vi "MT Detect ASK.vi"(5 "input complex waveform":T3={"t0"=0.0, "dt"=1.0, "Y"=[]} {"Y" format="%.3f"; "dt" format="%^.2e"; "t0" format="%.4f"}, 7 "ASK system parameters":T2={"samples per symbol (16)"=16, "symbol map"=[]} {"symbol map" format="%.3f"}, 9 "synchronization parameters":T1 {"sync sequence" format="%.2f"}, 11 "error in (no error)":errorcluster, 12 "matched filter coefficients":dbl[](array[numeric]) format="%.2f", 13 "reset? (T)":bool=TRUE, 14 "flush buffers? (F)":bool) -> (6 "output bit stream":i8[](array[numeric]), 10 "sync found index (symbols)":dbl format="%.4f", 15 "error out":errorcluster)   [LabVIEW 2020, in "niDMT.lvlib"]
doc: "Demodulates an amplitude-shift keying (ASK)-modulated complex baseband waveform and returns the demodulated bit stream. This VI attempts to remove carrier and phase offset by locking to the carrier signal."
uses:
  <vilib>/addons/Modulation/niDMT.lvlib
  <vilib>/addons/Modulation/Analog/controls/Complex Data Waveform.ctl
  <vilib>/Utility/error.llb/Error Cluster From Error Code.vi
  <vilib>/addons/Modulation/Digital/Support/Common/mod_Truncate FIR Filter (complex).vi
  <vilib>/addons/Modulation/niAMT.lvlib
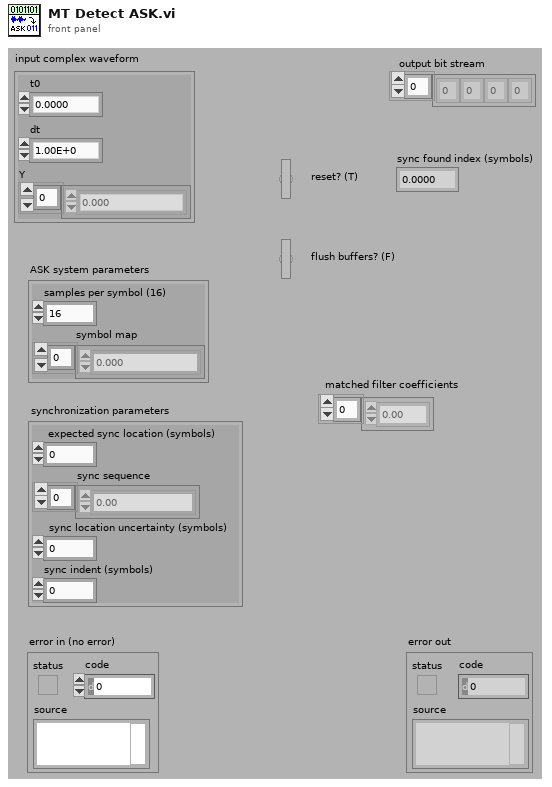
[diagram p1: front panel]
types:
  T1 = cluster{"expected sync location (symbols)":i32, "sync sequence":cdb[], "sync location uncertainty (symbols)":i32, "sync indent (symbols)":i32}
  T2 = cluster{"samples per symbol (16)":i32, "symbol map":cdb[]}
  T3 = typedef "niAMT.lvlib/Complex Data Waveform.ctl" = cluster{"t0":dbl, "dt":dbl, "Y":cdb[]}
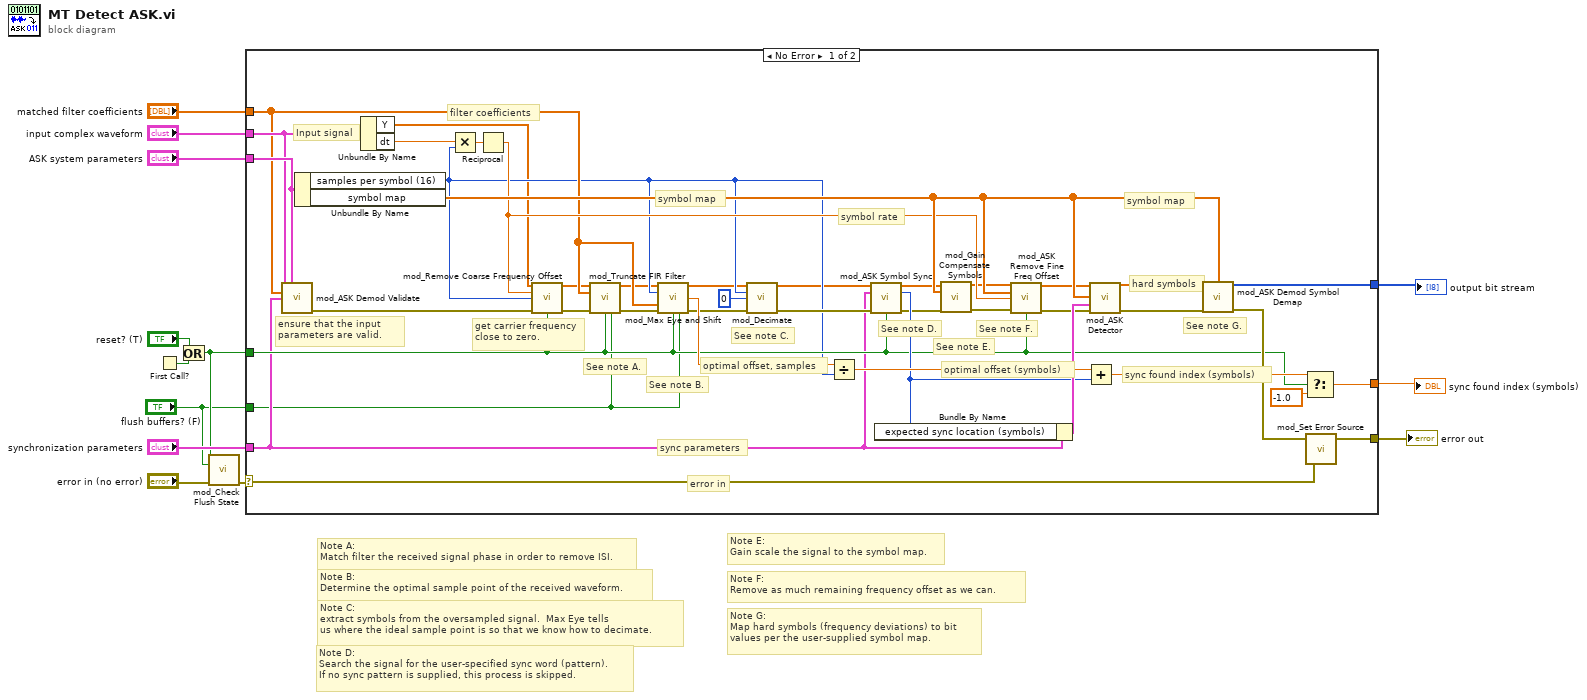
[diagram p0: block diagram]
diagram:
  # "Note E:\nGain scale the signal to the symbol map."
  # "Note G:\nMap hard symbols (frequency deviations) to bit\nvalues per the user-supplied symbol map."
  # "Note D:\nSearch the signal for the user-specified sync word (pattern).\nIf no sync pattern is supplied, this process is skipped."
  # "Note F:\nRemove as much remaining frequency offset as we can."
  # "Note C:\nextract symbols from the oversampled signal.  Max Eye tells\nus where the ideal sample point is so that we know how to decimate."
  # "Note B:\nDetermine the optimal sample point of the received waveform."
  # "Note A:\nMatch filter the received signal phase in order to remove ISI."
  n1 = First Call?() -> (First Call?: T/F=w6:bool)
  n2 = Or(x="reset? (T)", y=w6) -> (x .or. y?=w2:bool)
  n3 = call <vilib>:"mod_Check Flush State.vi"("reset?"=w2, "flush buffers? (F)"="flush buffers? (F)", "error in (no error)"="error in (no error)") -> ("error out"=w4:errorcluster)  [unwired: 12 out]
  n4 = case shown="No Error" w4 {
    selector: w4 -> [w35 w55]
    tunnel: w2 -> [w28 _]
    tunnel: "input complex waveform" -> [w39 _]
    tunnel: [w34 w55] -> w7
    tunnel: "matched filter coefficients" -> [w25 _]
    tunnel: [w54 _] -> w9
    tunnel: [w40 _] -> w8
    tunnel: "ASK system parameters" -> [w51 _]
    tunnel: "synchronization parameters" -> [w22 _]
    tunnel: "flush buffers? (F)" -> [w21 _]
    frame No Error {
      # "filter coefficients"
      # "error in"
      # "Input signal"
      # "sync found index (symbols)"
      # "symbol rate"
      # "hard symbols"
      # "symbol map"
      # "sync parameters"
      # "error in"
      # "symbol map"
      # "See note E."
      # "See note G."
      # "See note D."
      # "See note F."
      # "See note C."
      # "get carrier frequency close to zero."
      # "ensure that the input parameters are valid."
      # "See note B."
      # "See note A."
      # "optimal offset (symbols)"
      # "optimal offset, samples"
      n5 = call <vilib>:"mod_ASK Demod Validate.vi"("Input Complex Waveform"=w39, "PAM System Parameters"=w51, "Matched Filter Coefficients"=w25, "Synchronization Parameters"=w22) -> ("error out"=w45:errorcluster)  [unwired: 11 out]
      n6 = Unbundle By Name(w51) -> ("samples per symbol (16)"=w23:i32, "symbol map"=w31:cdb[])
      n7 = Unbundle By Name(w39) -> ("Y"=w20:cdb[], "dt"=w48:dbl)
      n8 = Multiply(x=w48, y=w23) -> (x*y=w49:dbl)
      n9 = Reciprocal(x=w49) -> (1/x=w29:dbl)
      n10 = call <vilib>:"mod_Remove Coarse Frequency Offset.vi"("Signal In"=w20, "Symbol Rate, Hz"=w29, "Samples Per Symbol (16)"=w23, "error in (no error)"=w45, "Reset? (T)"=w28) -> ("Signal Out"=w19:cdb[], "error out"=w53:errorcluster)  [unwired: 9 out]
      n11 = call-poly <vilib>:"mod_Truncate FIR Filter.vi"("Signal In"=w19, "Filter Coefficients"=w25, "error in (no error)"=w53, "Reset? (T)"=w28, "flush buffers? (F)"=w21) -> ("Signal Out"=w18:cdb[], "error out"=w46:errorcluster)  [unwired: 7 in, 2 out]
      n12 = call <vilib>:"mod_Max Eye and Shift.vi"("Signal In"=w18, "Samples Per Symbol (16)"=w23, "matched filter coefficients"=w25, "error in (no error)"=w46, "Reset? (T)"=w28, "flush buffers? (F)"=w21) -> ("Signal Out"=w17:cdb[], "Optimal Offset (in Samples)"=w38:dbl, "error out"=w24:errorcluster)  [unwired: 1 in, 6 out]
      n13 = call <vilib>:"mod_Decimate.vi"("Signal In"=w17, "Samples Per Symbol (16)"=w23, "Offset"=0, "error in (no error)"=w24) -> ("Signal Out"=w16:cdb[], "error out"=w50:errorcluster)  [unwired: 1 in, 9 out]
      n14 = Divide(x=w38, y=w23) -> (x/y=w47:dbl)
      n15 = call <vilib>:"mod_ASK Symbol Sync.vi"("Signal In"=w16, "Synchronization Parameters"=w22, "error in (no error)"=w50, "Reset? (T)"=w28) -> ("Signal Out"=w15:cdb[], "Sync Location (symbols)"=w44:i32, "error out"=w33:errorcluster)  [unwired: 9 out]
      n16 = Bundle By Name(cluster=w22, "expected sync location (symbols)"=w44) -> (w52:T1)
      n17 = call <vilib>:"mod_Gain Compensate Symbols.vi"("Symbols In"=w15, "Symbol Map"=w31, "error in (no error)"=w33) -> ("Symbols Out"=w14:cdb[], "error out"=w32:errorcluster)  [unwired: 11 out]
      n18 = call <vilib>:"mod_ASK Remove Fine Freq Offset.vi"("Symbols"=w14, "Symbol Map"=w31, "Symbol Rate, Hz"=w29, "error in (no error)"=w32, "Reset? (T)"=w28) -> ("Symbols"=w30:cdb[], "error out"=w43:errorcluster)  [unwired: 9 out]
      n19 = Add(x=w47, y=w44) -> (x+y=w41:dbl)
      n20 = call <vilib>:"mod_ASK Detector.vi"("Signal In"=w30, "Symbol Map"=w31, "Synchronization Parameters"=w52, "error in (no error)"=w43) -> ("Signal Out"=w26:cdb[], "error out"=w27:errorcluster)  [unwired: 10 out]
      n21 = call <vilib>:"mod_ASK Demod Symbol Demap.vi"("Symbols In"=w26, "Symbol Map"=w31, "error in (no error)"=w27) -> ("Bits Out"=w54:i8[], "error out"=w36:errorcluster)  [unwired: 1 in, 10 out]
      n22 = Select(t=w41, s=w28, f=-1.0) -> (s? t:f=w40:dbl)
      n23 = call <vilib>:"mod_Set Error Source.vi"("initial error in (no error)"=w35, "final error in (no error)"=w36) -> ("error out"=w34:errorcluster)  [unwired: 3 out]
    }
    frame Error {
    }
  }
  "error out" <- w7
  "sync found index (symbols)" <- w8
  "output bit stream" <- w9
